vi "FTW-XML-Query-ElementValue.vi"(0 "XML Node":refnum<k20>, 5 "XPath":string, 11 "error in":errorcluster) -> (4 "XML Node out":refnum<k20>, 6 "Value":string, 8 "Name":string, 10 "Found?":bool, 15 "error out":errorcluster)   [LabVIEW 2015]
uses:
  <resource>/objmgr/DOMUserDefRef.rc
panel:
  # "Inputs"
  # "Outputs"
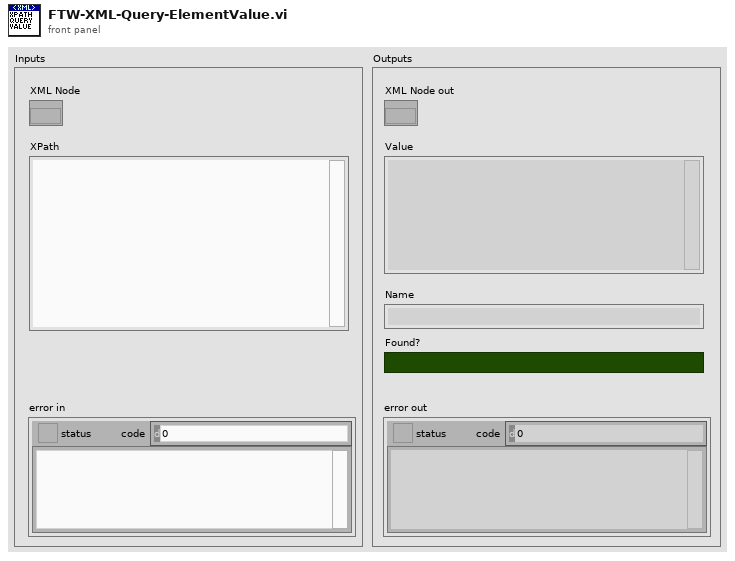
[diagram p1: front panel]
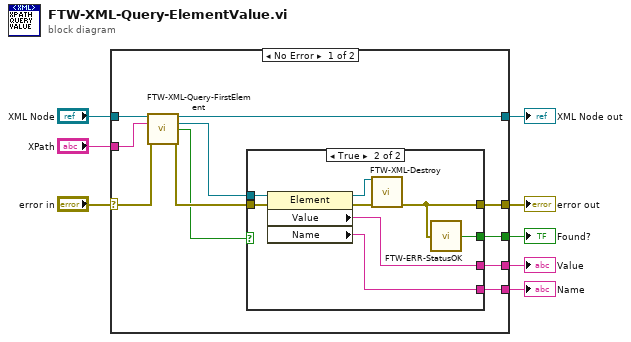
[diagram p0: block diagram]
diagram:
  n1 = case shown="No Error" "error in" {
    selector: "error in" -> [w13 w30]
    tunnel: [w19 w30] -> w8
    tunnel: "XML Node" -> [w15 w29]
    tunnel: [w16 w29] -> w5
    tunnel: "XPath" -> [w14 _]
    tunnel: [w18 _] -> w3
    tunnel: [w17 _] -> w2
    tunnel: [w9 _] -> w1
    frame No Error {
      n2 = call "FTW-XML-Query-FirstElement.vi"("XML Node"=w15, "XPath Query"=w14, "error in"=w13) -> ("XML Node out"=w16:refnum<k20>, "First Matched Element"=w10:refnum<k20>, "Found?"=w11:bool, "error out"=w12:errorcluster)  [unwired: 8 in, 1 out]
      n3 = case shown="True" w11 {
        tunnel: w12 -> [w20 w28]
        tunnel: [w20 w22] -> w19
        tunnel: [_ w27] -> w18
        tunnel: w10 -> [_ w26]
        tunnel: [_ w25] -> w17
        tunnel: [_ w21] -> w9
        frame False {
        }
        frame True {
          n4 = property class="Element"(reference=w26, error in=w28) -> (reference out=w24:refnum<k20>, error out=w23:errorcluster, "Value"=w27:string, "Name"=w21:string)
          n5 = call "FTW-XML-Destroy.vi"("XML Node"=w24, "error in"=w23) -> ("error out"=w22:errorcluster)  [unwired: 13 in]
          n6 = call "FTW-ERR-StatusOK.vi"("error to check"=w22) -> ("Status OK?"=w25:bool)
        }
      }
    }
    frame Error {
    }
  }
  "error out" <- w8
  "XML Node out" <- w5
  "Found?" <- w2
  "Value" <- w3
  "Name" <- w1
